vi "toStringArray.vi"(8 "error in (no error)":errorcluster, 11 "ScriptEventList in":refnum<class "ScriptEventList.lvclass">) -> (0 "error out":errorcluster, 2 "Array":string[][](array[string]), 3 "ScriptEventList out":refnum<class "ScriptEventList.lvclass">)   [LabVIEW 2009, in "Tools.lvlib" / "Scripting.lvlib" / "ScriptEventList.lvclass"]
uses:
  ScriptEventList.lvclass
  ScriptEventList.lvclass/ScriptEventList.ctl
  ScriptEvent.lvclass
  ScriptEvents/Ramp/RampEvent/RampEvent.lvclass
  ScriptEvents/RfRamp/RfRamp.lvclass
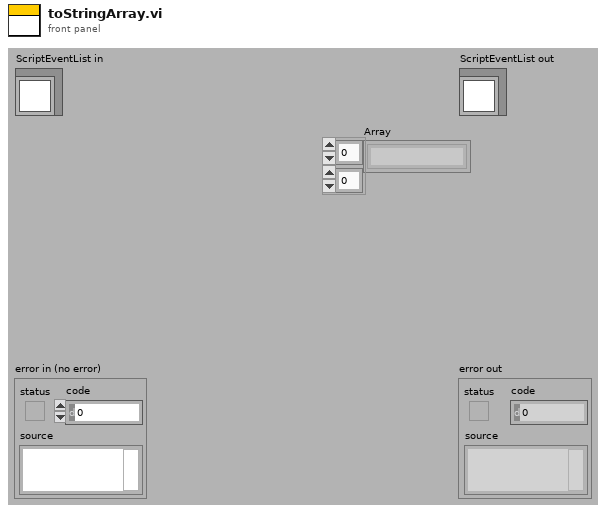
[diagram p1: front panel]
types:
  T1 = enum16{"changeValue", "pulse", "clock", "rampUp", "rampDown", "singleTone", "singleToneRamp", "playFile", "rf", "rfRamp", "delay"}
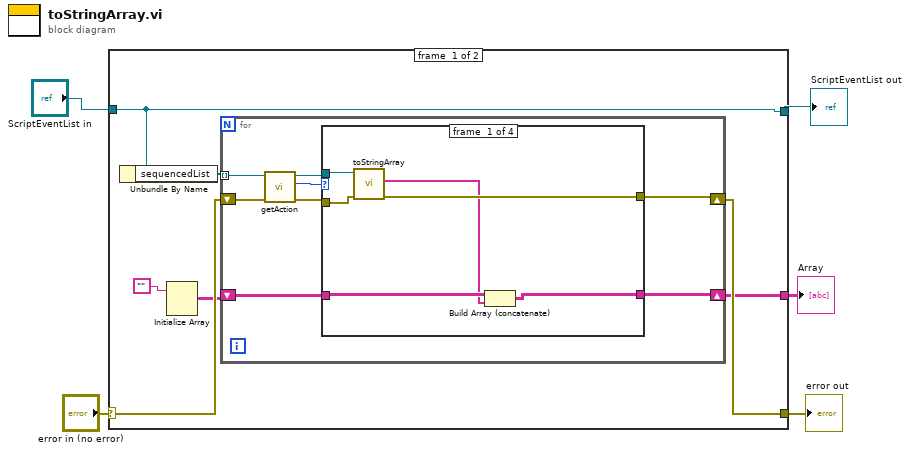
[diagram p0: block diagram]
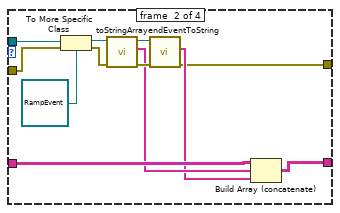
[diagram p2: hidden frame]
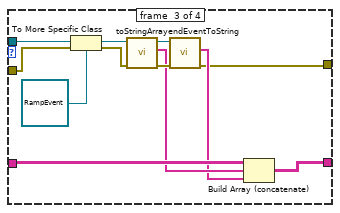
[diagram p3: hidden frame]
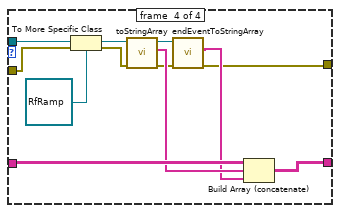
[diagram p4: hidden frame]
diagram:
  n1 = case shown="No Error" "error in (no error)" {
    selector: "error in (no error)" -> [w12 w64]
    tunnel: [w7 w64] -> w4
    tunnel: [w8 w63] -> w2
    tunnel: "ScriptEventList in" -> [w8 w63]
    tunnel: [w6 _] -> w1
    frame #0 {
      n2 = Unbundle By Name(w8) -> ("sequencedList"=w9:refnum<class "ScriptEvent.lvclass">[])
      n3 = Initialize Array("") -> (w11:string[][])  [unwired: 2 in]
      n4 = for {
        shift-right: [w16] -> w7
        shift-left: w12 -> [w17]
        shift-right: [w14] -> w6
        shift-left: w11 -> [w15]
        tunnel: w9 -> [w13] mode=indexing
        n5 = call "getAction.vi"("error in (no error)"=w17, "ScriptEvent.lvclass in"=w13) -> ("error out"=w18:errorcluster, "action"=w20:T1, "ScriptEvent.lvclass out"=w19:refnum<class "ScriptEvent.lvclass">)  [unwired: 7 in]
        n6 = case shown="\"changeValue\", Default" w20 {
          tunnel: w19 -> [w26 w37 w49 w62]
          tunnel: w18 -> [w25 w36 w48 w61]
          tunnel: [w24 w27 w39 w51] -> w16
          tunnel: w15 -> [w23 w31 w43 w58]
          tunnel: [w22 w28 w42 w57] -> w14
          frame #0 {
            n7 = call-dynamic "toStringArray.vi"("error in (no error)"=w25, "ScriptEvent in"=w26) -> ("error out"=w24:errorcluster, "eventStringArray"=w21:string[])  [unwired: 7 in, 1 out]
            n8 = Build Array (concatenate)(w23, w21) -> (w22:string[][])
          }
          frame #1 {
            n9 = To More Specific Class(target class=refnum<class "RampEvent.lvclass"> refnum ("Tools.lvlib:Scripting.lvlib:RampEvent.lvclass"), reference=w37, error in=w36) -> (specific class reference=w35:refnum<class "RampEvent.lvclass">, error out=w34:errorcluster)
            n10 = call-dynamic "toStringArray.vi"("error in (no error)"=w34, "RampEvent in"=w35) -> ("error out"=w33:errorcluster, "eventStringArray"=w30:string[], "RampEvent out"=w32:refnum<class "RampEvent.lvclass">)  [unwired: 7 in]
            n11 = call "endEventToString.vi"("error in (no error)"=w33, "RampEvent in"=w32) -> ("error out"=w27:errorcluster, "eventStringArray"=w29:string[])  [unwired: 7 in, 1 out]
            n12 = Build Array (concatenate)(w31, w30, w29) -> (w28:string[][])
          }
          frame #2 {
            n13 = To More Specific Class(target class=refnum<class "RampEvent.lvclass"> refnum ("Tools.lvlib:Scripting.lvlib:RampEvent.lvclass"), reference=w49, error in=w48) -> (specific class reference=w46:refnum<class "RampEvent.lvclass">, error out=w45:errorcluster)
            n14 = call-dynamic "toStringArray.vi"("error in (no error)"=w45, "RampEvent in"=w46) -> ("error out"=w44:errorcluster, "eventStringArray"=w41:string[], "RampEvent out"=w47:refnum<class "RampEvent.lvclass">)  [unwired: 7 in]
            n15 = call "endEventToString.vi"("error in (no error)"=w44, "RampEvent in"=w47) -> ("error out"=w39:errorcluster, "eventStringArray"=w40:string[])  [unwired: 7 in, 1 out]
            n16 = Build Array (concatenate)(w43, w41, w40) -> (w42:string[][])
          }
          frame #3 {
            n17 = To More Specific Class(target class=refnum<class "RfRamp.lvclass"> refnum ("Tools.lvlib:Scripting.lvlib:RfRamp.lvclass"), reference=w62, error in=w61) -> (specific class reference=w60:refnum<class "RfRamp.lvclass">, error out=w59:errorcluster)
            n18 = call-dynamic "toStringArray.vi"("error in (no error)"=w59, "RfRamp in"=w60) -> ("error out"=w53:errorcluster, "eventStringArray"=w56:string[], "RfRamp out"=w54:refnum<class "RfRamp.lvclass">)  [unwired: 7 in]
            n19 = call "endEventToStringArray.vi"("error in (no error)"=w53, "RfRamp in"=w54) -> ("error out"=w51:errorcluster, "eventStringArray"=w52:string[])  [unwired: 7 in, 1 out]
            n20 = Build Array (concatenate)(w58, w56, w52) -> (w57:string[][])
          }
        }
      }
    }
    frame #1 {
    }
  }
  "error out" <- w4
  "ScriptEventList out" <- w2
  "Array" <- w1
